vi "KINECT_Axis_Convert.vi"(8 "Arm Drive Min (Reverse)":dbl, 9 "Skeleton Vertices":cluster{"x":sgl, "y":sgl, "z":sgl}[](array[cluster]), 10 "Wrist Input":T1 items=["HipCenter", "Spine", "ShoulderCenter", "Head", "ShoulderLeft", "ElbowLeft", "WristLeft", "HandLeft", "ShoulderRight", "ElbowRight", "WristRight", "HandRight", "HipLeft", "KneeLeft", "AnkleLeft", "FootLeft", "HipRight", "KneeRight", "AnkleRight", "FootRight"], 11 "Arm Drive Max (Forward)":dbl) -> (1 "Z Axis Out":sgl, 2 "Punch Output (-1 to 1)":dbl, 3 "In Range ?":bool)   [LabVIEW 2011]
uses:
  <vilib>/addons/Kinect/Skeleton Vertex Index.ctl
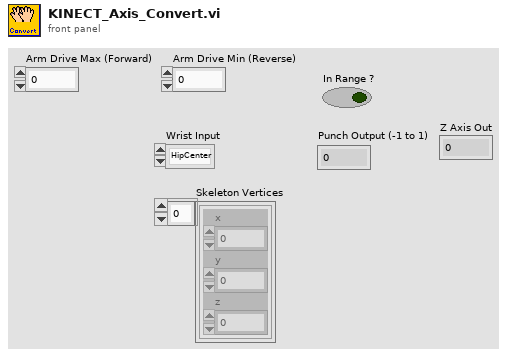
[diagram p1: front panel]
types:
  T1 = typedef "Skeleton Vertex Index.ctl" = i32
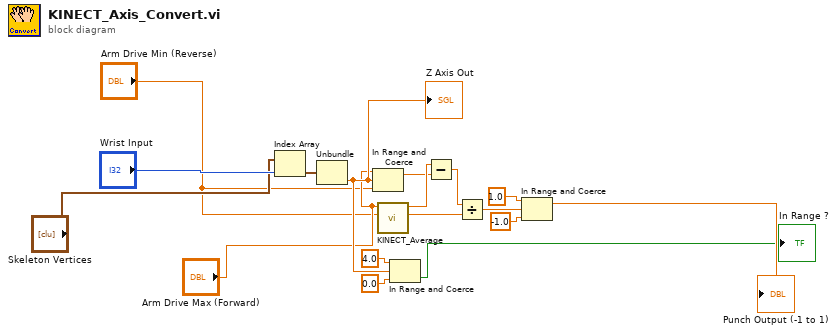
[diagram p0: block diagram]
diagram:
  n1 = Index Array(array="Skeleton Vertices", index="Wrist Input") -> (element=w8:cluster{"x":sgl, "y":sgl, "z":sgl})
  n2 = Unbundle(w8) -> ("z"=w17:sgl)  [unwired: 2 out]
  "Z Axis Out" <- w17
  n3 = In Range and Coerce(upper limit="Arm Drive Max (Forward)", x=w17, lower limit="Arm Drive Min (Reverse)") -> (coerced(x)=w10:dbl)  [unwired: 1 out]
  n4 = call "KINECT_Average.vi"("Min"="Arm Drive Min (Reverse)", "Max"="Arm Drive Max (Forward)") -> ("Range/2"=w12:dbl, "Average"=w11:dbl)  [unwired: 8 in]
  n5 = In Range and Coerce(upper limit=4.0, x=w17, lower limit=0.0) -> (In Range?=→"In Range ?":bool)  [unwired: 1 out]
  n6 = Subtract(x=w11, y=w10) -> (x-y=w9:dbl)
  n7 = Divide(x=w9, y=w12) -> (x/y=w13:dbl)
  n8 = In Range and Coerce(upper limit=1.0 ("y"), x=w13, lower limit=-1.0 ("y")) -> (coerced(x)=→"Punch Output (-1 to 1)":dbl)  [unwired: 1 out]
